vi "HelioScan_3.vi"() -> ()   [LabVIEW 2010]
uses:
  labview_source/controls/update_picture.ctl
  common/xcontrols/XUserDropdown/XUserDropdown/XUserDropdown.xctl
  tools/HelioUpdateMH100803/HelioUpdateMH100803/HelioUpdateMH100803.lvclass
  common/classes/ErrorController/ErrorController/ErrorController.lvclass
  labview_source/type_definitions/clusters/controls_refs.ctl
  components/DAQ/GenericDAQ/GenericDAQ/GenericDAQ.lvclass
  components/ImageAssembler/GenericImageAssembler/GenericImageAssembler/GenericImageAssembler.lvclass
  components/DataCollection/GenericDataCollection/GenericDataCollection/GenericDataCollection.lvclass
  components/Display/GenericDisplay/GenericDisplay/GenericDisplay.lvclass
  components/Analyser/GenericAnalyser/GenericAnalyser/GenericAnalyser.lvclass
  components/ImagingMode/GenericImagingMode/GenericImagingMode/GenericImagingMode.lvclass
  components/Instrument/GenericInstrument/GenericInstrument/GenericInstrument.lvclass
  components/ScanHead/GenericScanHead/GenericScanHead/GenericScanHead.lvclass
  components/Stimulator/GenericStimulator/GenericStimulator/GenericStimulator.lvclass
  components/ExperimentController/GenericExperimentController/GenericExperimentController/GenericExperimentController.lvclass
  components/Stage/GenericStage/GenericStage/GenericStage.lvclass
  <vilib>/Utility/miscctls.llb/LVPointTypeDef.ctl
  components/DataCollection/GenericDataCollection/GenericDataCollection/trigger_enum.ctl
  common/classes/GenericComponent/GenericComponent/GenericComponent.lvclass
  <vilib>/Platform/browser.llb/Open URL in Default Browser (string).vi
  common/classes/ErrorController/ErrorController/class_data.vi
panel:
  in  "button:start_experiment":bool
  in  "button:start_single_sweep":bool
  in  "button:start_focus":bool
  out "saving message":string
  out "progress slider":u8(slide) caption="slider" scale=0.0..11.0
  in  "user":string(xcontrol)
  out "update icon":T1
  in  "file base name":string
  in  "data folder path":path
  in  "notebook":string caption="Notebook"
  in  "exit_button":bool
  in  "objective":string(combo)
  in  "save button":bool
  in  "settings tab":T2(tab)
  in  "imaging mode":string(combo)
  in  "experimental protocol":string(combo)
  in  "stimulator enabled?":bool
  in  "button: task manager":bool
  out "error handler":bool caption="error controller"
  out "experiment controller":bool
  out "imaging mode":bool
  out "scan head":bool
  out "DAQ":bool
  out "image assembler":bool
  out "data collection":bool
  out "display":bool
  out "analyser":bool
  out "stage":bool
  out "stimulator":bool
  out "instrument":bool
  out "Message":string="No Error"
  in  "title":bool caption="HelioScan 3.4.0.23d214112d"
  # "Note: stimulator only works in \"single sweep mode\" and \"experiment mode\"!"
  # "Loaded"
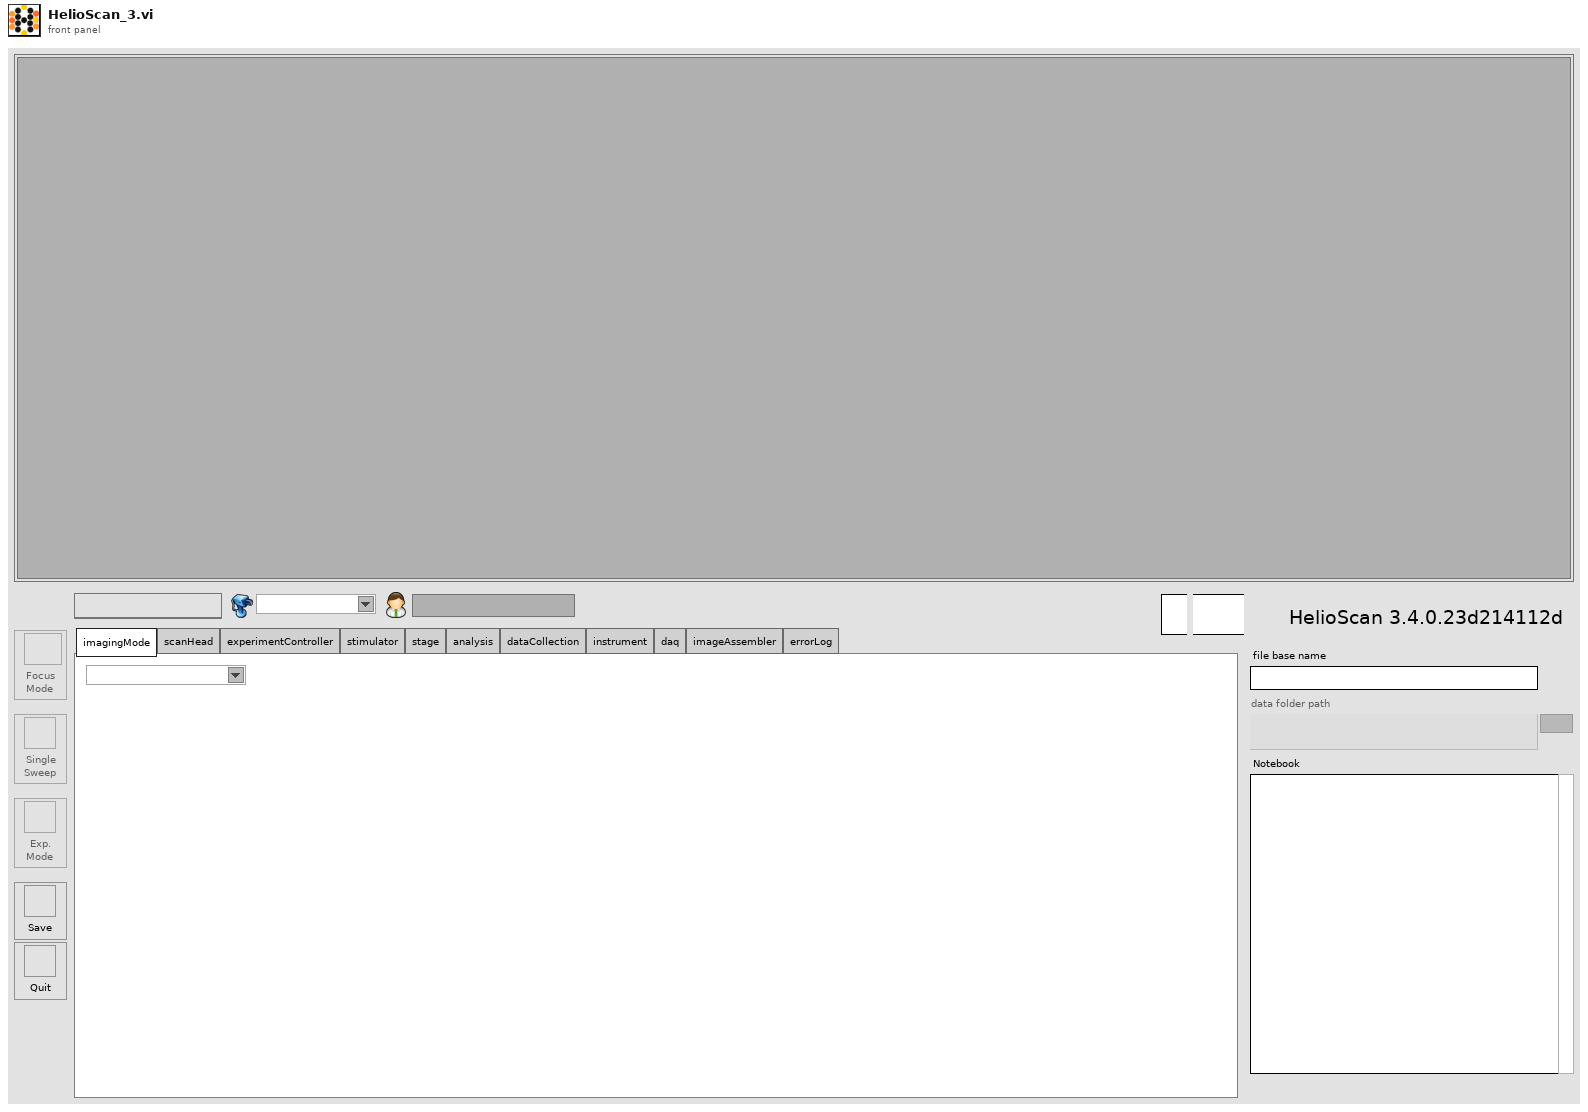
[diagram p1: front panel]
types:
  T1 = typedef "HelioUpdateMH100803.lvclass/update_picture.ctl" = u16
  T2 = enum32{"imagingMode", "scanHead", "experimentController", "stimulator", "stage", "analysis", "dataCollection", "instrument", "daq", "imageAssembler", "errorLog"}
  T3 = typedef "controls_refs.ctl" = cluster{"buttons":cluster{"start_focus":refnum<vi>, "start_single_sweep":refnum<vi>, "start_experiment":refnum<vi>, "save":refnum<vi>, "exit":refnum<vi>}, "tabs":cluster{"main":refnum<vi>, "settings":refnum<vi>}, "subpanels":cluster{"imagingMode":refnum<vi>, "scanHead":refnum<vi>, "display":refnum<vi>, "experimentController":refnum<vi>, "instrument":refnum<vi>, "stage":refnum<vi>, "stimulator":refnum<vi>, "dataCollection":refnum<vi>, "analyser":refnum<vi>, "daq":refnum<vi>, "imageAssembler":refnum<vi>}, "drop-downs":cluster{"imagingMode":refnum<vi>, "experimentalController":refnum<vi>, "objective":refnum<vi>}, "status lights":cluster{"experimentController":refnum<vi>, "imagingMode":refnum<vi>, "scanHead":refnum<vi>, "daq":refnum<vi>, "imageAssembler":refnum<vi>, "dataCollection":refnum<vi>, "display":refnum<vi>, "analyser":refnum<vi>, "stage":refnum<vi>, "stimulator":refnum<vi>, "instrument":refnum<vi>}, "message":refnum<vi>, "stimulator enabled?":refnum<vi>, "saving":cluster{"data folder path":refnum<vi>, "file base name":refnum<vi>, "notebook":refnum<vi>}, "progress bar":refnum<vi>, "update icon":refnum<vi>, "title":refnum<vi>, "main vi":refnum<vi>, "user":refnum<vi>}
  T4 = typedef "LVPointTypeDef.ctl" = cluster{"Horizontal":i16, "Vertical":i16}
  T5 = typedef "GenericDataCollection.lvclass/trigger_enum.ctl" = enum16{"NULL", "save", "reset"}
  T6 = enum8{"Enabled", "Disabled", "Disabled and Grayed Out"}
  T7 = enum32{"Invalid", "Standard", "Closed", "Hidden", "Minimized", "Maximized"}
  T8 = enum16{"focus mode", "single sweep mode", "experiment mode"}
  T9 = typedef "main_trigger_enum.ctl" = enum16{"NULL", "initialise", "terminate", "start", "stop", "change objective", "change experimentController", "change imagingMode", "save notebook", "started saving", "finished saving", "expCtr ready", "expCtr missing", "imgMd ready", "imgMd missing", "scanHd ready", "scanHd missing", "DAQ ready", "DAQ missing", "imgAsm ready", "imgAsm missing", "dataColl ready", "dataColl missing", "display ready", "display missing", "analysr ready", "analysr missing", "instrmnt ready", "instrmnt missing", "stimltr ready", "stimltr missing", "stage ready", "stage missing"}
  T10 = typedef "run_mode_enum.ctl" = enum16{"focus mode", "single sweep mode", "experiment mode"}
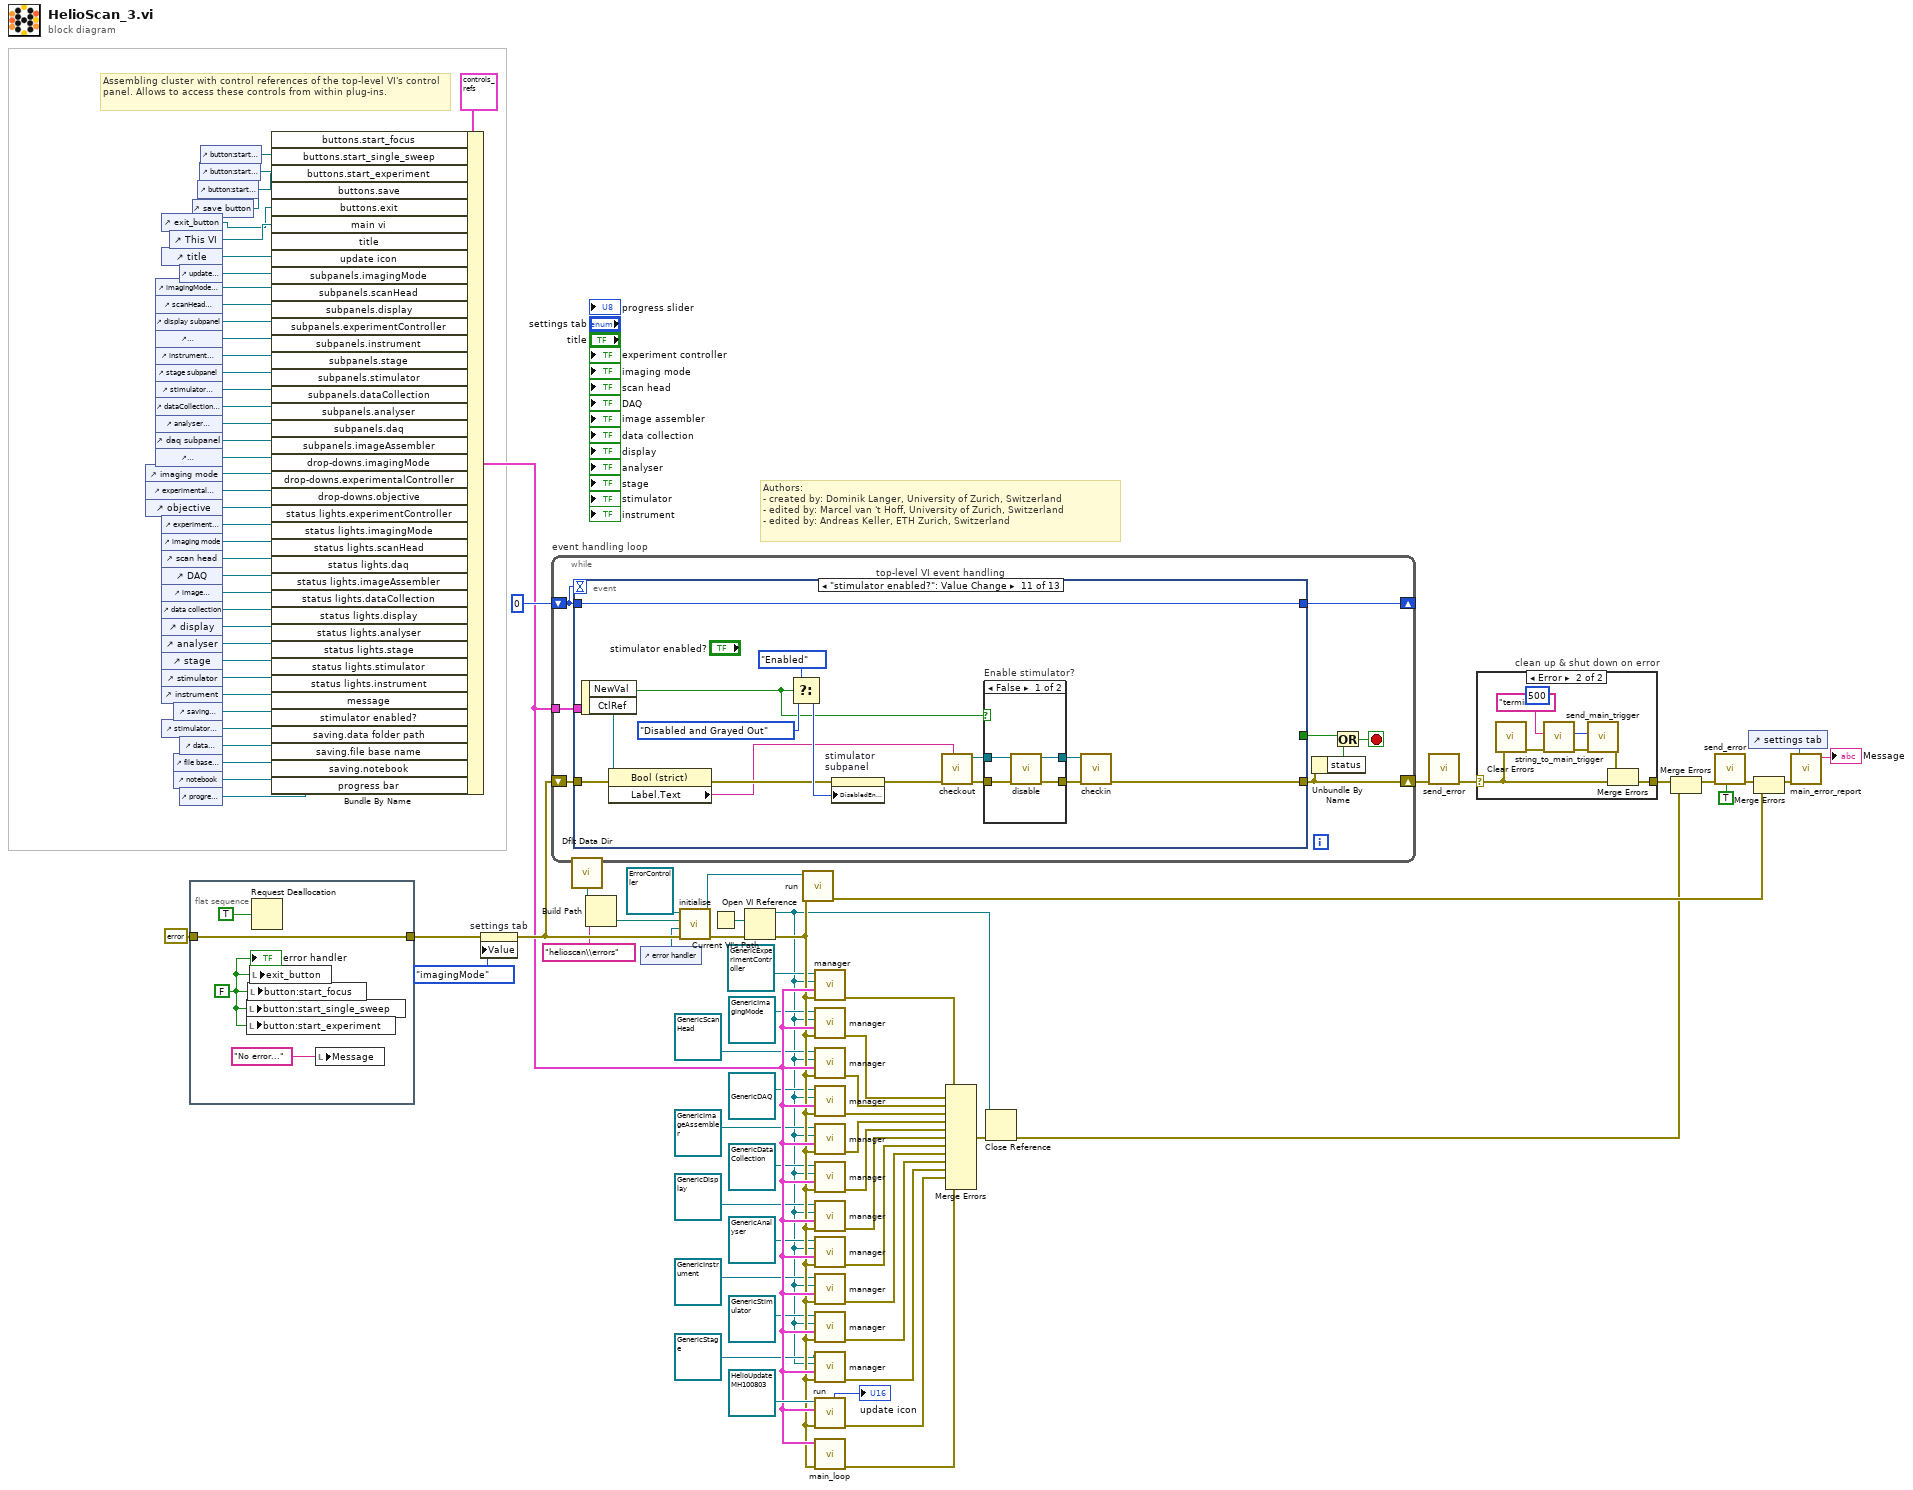
[diagram p0: block diagram]
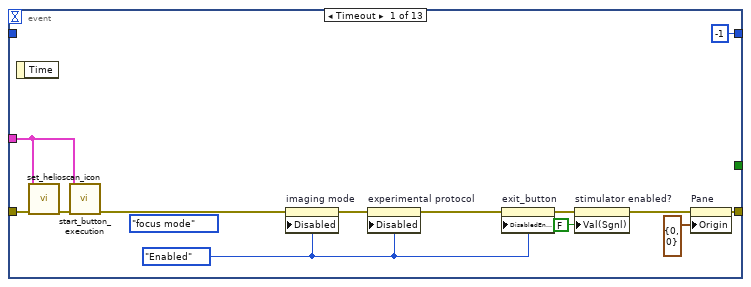
[diagram p3: hidden frame]
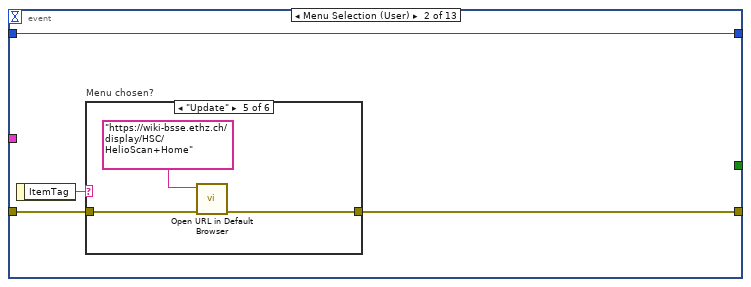
[diagram p4: hidden frame]
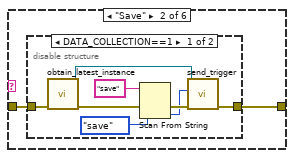
[diagram p6: hidden frame]
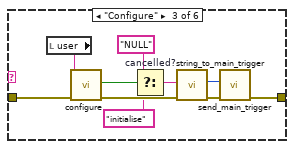
[diagram p8: hidden frame]
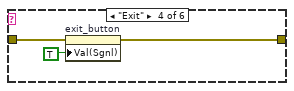
[diagram p9: hidden frame]
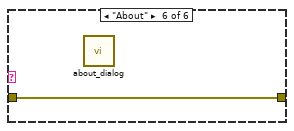
[diagram p10: hidden frame]
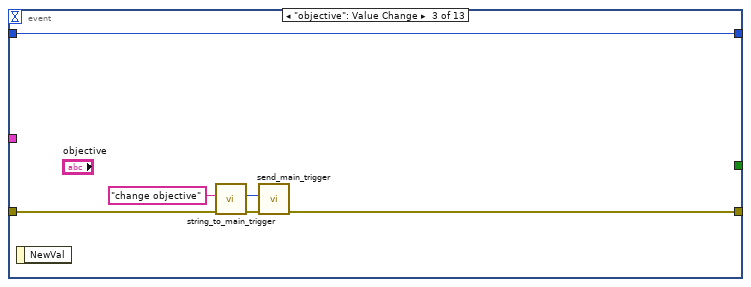
[diagram p11: hidden frame]
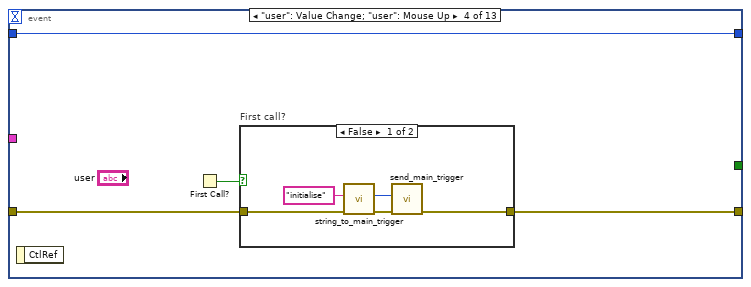
[diagram p12: hidden frame]
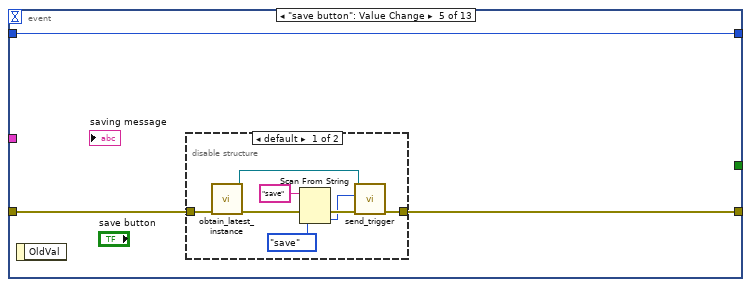
[diagram p14: hidden frame]
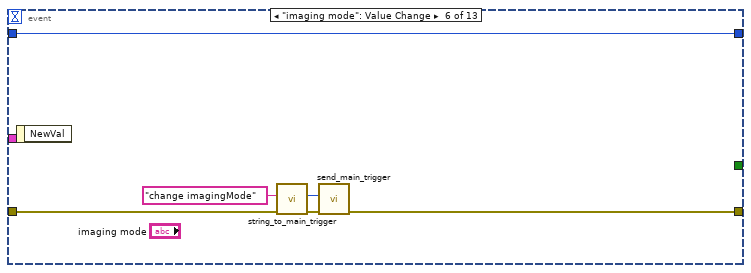
[diagram p16: hidden frame]
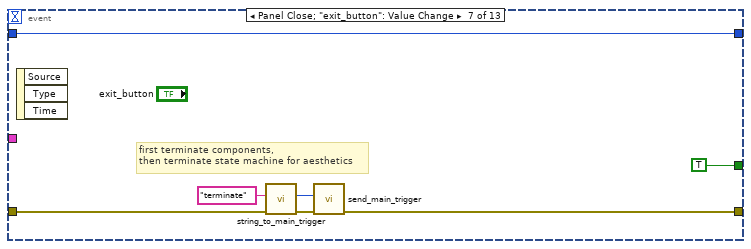
[diagram p17: hidden frame]
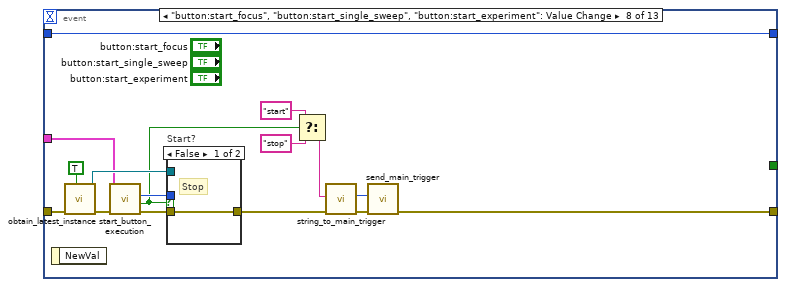
[diagram p18: hidden frame]
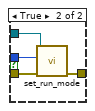
[diagram p19: hidden frame]
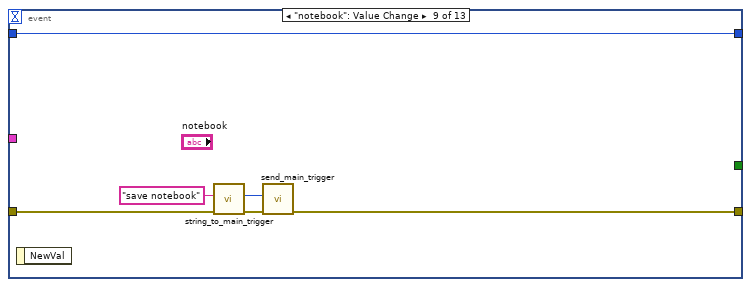
[diagram p20: hidden frame]
diagram:
  # "Authors: \n- created by: Dominik Langer, University of Zurich, Switzerland\n- edited by: Marcel van 't Hoff, University of Zurich, Switzerland\n- edited by: Andreas Keller, ETH Zurich, Switzerland"
  # "Assembling cluster with control references of the top-level VI's control panel. Allows to access these controls from within plug-ins."
  n1 = control-ref of="imaging mode"() -> (w83:refnum<vi>)
  n2 = control-ref of="experimental protocol"() -> (w84:refnum<vi>)
  n3 = control-ref of="objective"() -> (w69:refnum<vi>)
  n4 = control-ref of="imagingMode subpanel"() -> (w63:refnum<vi>)
  n5 = control-ref of="scanHead subpanel"() -> (w94:refnum<vi>)
  n6 = control-ref of="display subpanel"() -> (w90:refnum<vi>)
  n7 = control-ref of="experimentController subpanel"() -> (w91:refnum<vi>)
  n8 = control-ref of="instrument subpanel"() -> (w89:refnum<vi>)
  n9 = control-ref of="stage subpanel"() -> (w87:refnum<vi>)
  n10 = control-ref of="stimulator subpanel"() -> (w86:refnum<vi>)
  n11 = control-ref of="dataCollection subpanel"() -> (w85:refnum<vi>)
  n12 = control-ref of="analyser subpanel"() -> (w82:refnum<vi>)
  n13 = control-ref of="daq subpanel"() -> (w61:refnum<vi>)
  n14 = control-ref of="imageAssembler subpanel"() -> (w62:refnum<vi>)
  n15 = control-ref of="exit_button"() -> (w1:refnum<vi>)
  n16 = control-ref of="title"() -> (w44:refnum<vi>)
  n17 = control-ref of="experiment controller"() -> (w73:refnum<vi>)
  n18 = control-ref of="imaging mode"() -> (w72:refnum<vi>)
  n19 = control-ref of="scan head"() -> (w76:refnum<vi>)
  n20 = control-ref of="DAQ"() -> (w75:refnum<vi>)
  n21 = control-ref of="image assembler"() -> (w74:refnum<vi>)
  n22 = control-ref of="data collection"() -> (w71:refnum<vi>)
  n23 = control-ref of="display"() -> (w77:refnum<vi>)
  n24 = control-ref of="analyser"() -> (w78:refnum<vi>)
  n25 = control-ref of="stage"() -> (w81:refnum<vi>)
  n26 = control-ref of="stimulator"() -> (w80:refnum<vi>)
  n27 = control-ref of="instrument"() -> (w70:refnum<vi>)
  n28 = control-ref of="stimulator enabled?"() -> (w67:refnum<vi>)
  n29 = control-ref of="This VI"() -> (w41:refnum<vi>)
  n30 = control-ref of="saving message"() -> (w45:refnum<vi>)
  n31 = control-ref of="file base name"() -> (w65:refnum<vi>)
  n32 = control-ref of="notebook"() -> (w64:refnum<vi>)
  n33 = control-ref of="update icon"() -> (w43:refnum<vi>)
  n34 = control-ref of="data folder path"() -> (w66:refnum<vi>)
  n35 = control-ref of="progress bar"() -> (w49:refnum<vi>)
  n36 = flat-sequence {
    tunnel: errorcluster {"status"=FALSE, "code"=0, "source"=""} ("error in (no error)") -> [w98]
    tunnel: [w98] -> w7
    frame #0 {
      w95 = FALSE
      n37 = local write "button:start_single_sweep"(w95) -> ()
      n38 = local write "button:start_experiment"(w95) -> ()
      n39 = local write "button:start_focus"(w95) -> ()
      n40 = local write "exit_button"(w95) -> ()
      n41 = Request Deallocation(TRUE ("flag")) -> ()
      n42 = local write "Message"("No error...") -> ()
      "error handler" <- w95
    }
  }
  n43 = control-ref of="save button"() -> (w2:refnum<vi>)
  n44 = control-ref of="button:start_experiment"() -> (w3:refnum<vi>)
  n45 = control-ref of="button:start_single_sweep"() -> (w4:refnum<vi>)
  n46 = control-ref of="button:start_focus"() -> (w5:refnum<vi>)
  n47 = Bundle By Name(cluster=T3 {"buttons"={"start_focus"=refnum, "start_single_sweep"=refnum, "start_experiment"=refnum, "save"=refnum, "exit"=refnum}, "tabs"={"main"=refnum, "settings"=refnum}, "subpanels"={"imagingMode"=refnum, "scanHead"=refnum, "display"=refnum, "experimentController"=refnum, "instrument"=refnum, "stage"=refnum, "stimulator"=refnum, "dataCollection"=refnum, "analyser"=refnum, "daq"=refnum, "imageAssembler"=refnum}, "drop-downs"={"imagingMode"=refnum, "experimentalController"=refnum, "objective"=refnum}, "status lights"={"experimentController"=refnum, "imagingMode"=refnum, "scanHead"=refnum, "daq"=refnum, "imageAssembler"=refnum, "dataCollection"=refnum, "display"=refnum, "analyser"=refnum, "stage"=refnum, "stimulator"=refnum, "instrument"=refnum}, "message"=refnum, "stimulator enabled?"=refnum, "saving"={"data folder path"=refnum, "file base name"=refnum, "notebook"=refnum}, "progress bar"=refnum, "update icon"=refnum, "title"=refnum, "main vi"=refnum, "user"=refnum} ("control references"), "buttons.start_focus"=w5, "buttons.start_single_sweep"=w4, "buttons.start_experiment"=w3, "buttons.save"=w2, "buttons.exit"=w1, "main vi"=w41, "title"=w44, "update icon"=w43, "subpanels.imagingMode"=w63, "subpanels.scanHead"=w94, "subpanels.display"=w90, "subpanels.experimentController"=w91, "subpanels.instrument"=w89, "subpanels.stage"=w87, "subpanels.stimulator"=w86, "subpanels.dataCollection"=w85, "subpanels.analyser"=w82, "subpanels.daq"=w61, "subpanels.imageAssembler"=w62, "drop-downs.imagingMode"=w83, "drop-downs.experimentalController"=w84, "drop-downs.objective"=w69, "status lights.experimentController"=w73, "status lights.imagingMode"=w72, "status lights.scanHead"=w76, "status lights.daq"=w75, "status lights.imageAssembler"=w74, "status lights.dataCollection"=w71, "status lights.display"=w77, "status lights.analyser"=w78, "status lights.stage"=w81, "status lights.stimulator"=w80, "status lights.instrument"=w70, "message"=w45, "stimulator enabled?"=w67, "saving.data folder path"=w66, "saving.file base name"=w65, "saving.notebook"=w64, "progress bar"=w49) -> (w23:T3)
  n48 = property on="settings tab" class="TabCtl (strict)"(error in=w7, "Value"=T2."imagingMode" ("settings tab")) -> (error out=w35:errorcluster)  [unwired: 1 in, 1 out]
  n49 = while "event handling loop" {
    shift-right: [w104] -> _
    shift-left: 0 -> [w105]
    tunnel: w23 -> [w103]
    shift-right: [w102] -> w38
    shift-left: w35 -> [w106]
    stop <- w99 stop-if-true
    n50 = event "top-level VI event handling" shown="[10] \"stimulator enabled?\": Value Change" {
      selector: _ -> [_ _ _ _ _ _ _ _ _ _ _ _ _]
      dyn-events: _ -> [_ _ _ _ _ _ _ _ _ _ _ _ _]
      timeout: w105 -> [_ _ _ _ _ _ _ _ _ _ _ _ _]
      tunnel: [_ _ _ _ _ _ TRUE _ _ _ _ _ _] -> w101
      tunnel: [w117 w120 w157 w161 w170 w185 w191 w195 w219 w225 w234 w256 w262] -> w102
      tunnel: w106 -> [w110 w121 w156 w159 w169 w184 w187 w199 w218 w226 w232 w253 w273]
      tunnel: [-1 w123 w158 w162 w171 w186 w193 w209 w220 w228 w243 w257 w274] -> w104
      tunnel: w105 -> [_ w123 w158 w162 w171 w186 w193 w209 w220 w228 w243 w257 w274]
      tunnel: w103 -> [w108 _ _ _ _ _ _ w196 _ _ _ _ _]
      event Timeout {
        w114 = T6."Enabled" ("Disabled")
        (unwired) T8."focus mode" ("Value (Signaling)")
        n51 = event-data() -> ()  [unwired: 2 out]
        n52 = call "set_helioscan_icon.vi"("error in (no error)"=w110, "reference cluster in"=w108) -> ("error out"=w109:errorcluster)  [unwired: 9 in]
        n53 = call "start_button_execution.vi"("error in (no error)"=w109, "control references"=w108) -> ("error out"=w107:errorcluster)  [unwired: 7 in, 2 out]
        n54 = property on="imaging mode" class="CmbBox"(error in=w107, "Disabled"=w114) -> (error out=w118:errorcluster)  [unwired: 1 in, 1 out]
        n55 = property on="experimental protocol" class="CmbBox"(error in=w118, "Disabled"=w114) -> (error out=w115:errorcluster)  [unwired: 1 in, 1 out]
        n56 = property on="exit_button" class="Bool (strict)"(error in=w115, "DisabledEnum"=w114) -> (error out=w112:errorcluster)  [unwired: 1 in, 1 out]
        n57 = property on="stimulator enabled?" class="Bool (strict)"(error in=w112, "Val(Sgnl)"=FALSE ("stimulator enabled?")) -> (error out=w113:errorcluster)  [unwired: 1 in, 1 out]
        n58 = property on="Pane" class="Pane"(error in=w113, "Origin"=T4 {"Horizontal"=0, "Vertical"=0}) -> (error out=w117:errorcluster)  [unwired: 1 in, 1 out]
      }
      event Menu Selection (User) {
        n59 = event-data() -> ("ItemTag"=w122:string)  [unwired: 1 out]
        n60 = case "Menu chosen?" shown="\"Update\"" w122 {
          tunnel: w121 -> [w124 w126 w145 w148 w151 w152]
          tunnel: [w124 w125 w143 w146 w150 w152] -> w120
          frame Default {
          }
          frame "Save" {
            n61 = disable-structure shown="DATA_COLLECTION==1" {
              disable-tunnel: w126 -> [w133 w135]
              disable-tunnel: [w134 w135] -> w125
              frame condition #0 (active) {
                n62 = call "obtain_latest_instance.vi"("error in (no error)"=w133) -> ("error out"=w130:errorcluster, "GenericDataCollection out"=w132:refnum<class "GenericDataCollection.lvclass">)  [unwired: 1 in, 8 out]
                n63 = Scan From String(input string="save", error in=w130, default 1=trigger_enum."save" ("trigger")) -> (error out=w129:errorcluster, output 1=w128:T5)  [unwired: 2 in, 2 out]
                n64 = call-dynamic "send_trigger.vi"("error in (no error)"=w129, "trigger"=w128, "GenericDataCollection in"=w132) -> ("error out"=w134:errorcluster)  [unwired: 8 out]
              }
              frame condition #1 {
              }
            }
          }
          frame "Configure" {
            n65 = local read "user"() -> (w144:string)
            n66 = call "configure.vi"("error in (no error)"=w145, "user"=w144) -> ("error out"=w141:errorcluster, "cancelled?"=w142:bool)  [unwired: 1 in, 7 out]
            n67 = Select "cancelled?"(t="NULL", s=w142, f="initialise") -> (s? t:f=w137:string)
            n68 = call "string_to_main_trigger.vi"("error in (no error)"=w141, "trigger string"=w137) -> ("error out"=w140:errorcluster, "main trigger"=w136:T9)  [unwired: 8 in]
            n69 = call "send_main_trigger.vi"("error in (no error)"=w140, "trigger"=w136) -> ("error out"=w143:errorcluster)  [unwired: 9 in]
          }
          frame "Exit" {
            n70 = property on="exit_button" class="Bool (strict)"(error in=w148, "Val(Sgnl)"=TRUE) -> (error out=w146:errorcluster)  [unwired: 1 in, 1 out]
          }
          frame "Update" {
            n71 = call-poly <vilib>:"Open URL in Default Browser.vi"("error in (no error)"=w151, "URL"="https://wiki-bsse.ethz.ch/display/HSC/HelioScan+Home") -> ("error out"=w150:errorcluster)  [unwired: 4 in, 1 out]
          }
          frame "About" {
            n72 = call "about_dialog.vi"() -> ()  [unwired: 1 out]
          }
        }
      }
      event "objective": Value Change {
        n73 = event-data() -> ()  [unwired: 2 out]
        n74 = call "string_to_main_trigger.vi"("error in (no error)"=w156, "trigger string"="change objective") -> ("error out"=w155:errorcluster, "main trigger"=w154:T9)  [unwired: 8 in]
        n75 = call "send_main_trigger.vi"("error in (no error)"=w155, "trigger"=w154) -> ("error out"=w157:errorcluster)  [unwired: 9 in]
      }
      event "user": Value Change; "user": Mouse Up {
        n76 = event-data() -> ()  [unwired: 2 out]
        n77 = First Call?() -> (First Call?: T/F=w160:bool)
        n78 = case "First call?" shown="False" w160 {
          tunnel: [w167 w168] -> w161
          tunnel: w159 -> [w166 w168]
          frame False {
            n79 = call "string_to_main_trigger.vi"("error in (no error)"=w166, "trigger string"="initialise") -> ("error out"=w165:errorcluster, "main trigger"=w164:T9)  [unwired: 8 in]
            n80 = call "send_main_trigger.vi"("error in (no error)"=w165, "trigger"=w164) -> ("error out"=w167:errorcluster)  [unwired: 9 in]
          }
          frame True {
          }
        }
      }
      event "save button": Value Change {
        n81 = event-data() -> ()  [unwired: 2 out]
        n82 = disable-structure shown="default" {
          disable-tunnel: [w179 w180] -> w170
          disable-tunnel: w169 -> [w178 w180]
          frame condition #0 (active) {
            n83 = call "obtain_latest_instance.vi"("error in (no error)"=w178) -> ("error out"=w176:errorcluster, "GenericDataCollection out"=w177:refnum<class "GenericDataCollection.lvclass">)  [unwired: 1 in, 8 out]
            n84 = Scan From String(input string="save", error in=w176, default 1=trigger_enum."save" ("trigger")) -> (error out=w175:errorcluster, output 1=w173:T5)  [unwired: 2 in, 2 out]
            n85 = call-dynamic "send_trigger.vi"("error in (no error)"=w175, "trigger"=w173, "GenericDataCollection in"=w177) -> ("error out"=w179:errorcluster)  [unwired: 8 out]
          }
          frame condition #1 {
          }
        }
      }
      event "imaging mode": Value Change {
        n86 = event-data() -> ()  [unwired: 2 out]
        n87 = call "string_to_main_trigger.vi"("error in (no error)"=w184, "trigger string"="change imagingMode") -> ("error out"=w183:errorcluster, "main trigger"=w182:T9)  [unwired: 8 in]
        n88 = call "send_main_trigger.vi"("error in (no error)"=w183, "trigger"=w182) -> ("error out"=w185:errorcluster)  [unwired: 9 in]
      }
      event Panel Close; "exit_button": Value Change {
        # "first terminate components, \nthen terminate state machine for aesthetics"
        n89 = event-data() -> ()  [unwired: 4 out]
        n90 = call "string_to_main_trigger.vi"("error in (no error)"=w187, "trigger string"="terminate") -> ("error out"=w190:errorcluster, "main trigger"=w189:T9)  [unwired: 8 in]
        n91 = call "send_main_trigger.vi"("error in (no error)"=w190, "trigger"=w189) -> ("error out"=w191:errorcluster)  [unwired: 9 in]
      }
      event "button:start_focus", "button:start_single_sweep", "button:start_experiment": Value Change {
        n92 = event-data() -> ()  [unwired: 2 out]
        n93 = call "obtain_latest_instance.vi"("quick, but maybe outdated?"=TRUE, "error in (no error)"=w199) -> ("error out"=w198:errorcluster, "GenericScanMode out"=w208:refnum<class "GenericImagingMode.lvclass">)  [unwired: 8 out]
        n94 = call "start_button_execution.vi"("error in (no error)"=w198, "control references"=w196) -> ("error out"=w197:errorcluster, "start?"=w194:bool, "mode"=w200:T10)  [unwired: 7 in]
        n95 = case "Start?" shown="False" w194 {
          tunnel: w208 -> [_ w214]
          tunnel: [w210 w213] -> w201
          tunnel: w200 -> [_ w212]
          tunnel: w197 -> [w210 w211]
          frame False {
            # "Stop"
          }
          frame True {
            n96 = call-dynamic "set_run_mode.vi"("error in (no error)"=w211, "run mode"=w212, "GenericPlugin in"=w214) -> ("error out"=w213:errorcluster)  [unwired: 8 out]
          }
        }
        n97 = Select(t="start" ("trigger string"), s=w194, f="stop") -> (s? t:f=w203:string)
        n98 = call "string_to_main_trigger.vi"("error in (no error)"=w201, "trigger string"=w203) -> ("error out"=w205:errorcluster, "main trigger"=w206:T9)  [unwired: 8 in]
        n99 = call "send_main_trigger.vi"("error in (no error)"=w205, "trigger"=w206) -> ("error out"=w195:errorcluster)  [unwired: 9 in]
      }
      event "notebook": Value Change {
        n100 = event-data() -> ()  [unwired: 2 out]
        n101 = call "string_to_main_trigger.vi"("error in (no error)"=w218, "trigger string"="save notebook") -> ("error out"=w217:errorcluster, "main trigger"=w216:T9)  [unwired: 8 in]
        n102 = call "send_main_trigger.vi"("error in (no error)"=w217, "trigger"=w216) -> ("error out"=w219:errorcluster)  [unwired: 9 in]
      }
      event "file base name", "data folder path": Value Change {
        n103 = event-data() -> ()  [unwired: 2 out]
        n104 = call-dynamic "set_data_folder_path.vi"("error in (no error)"=w226, "data folder path"="data folder path", "GenericComponent in"=refnum<class "GenericComponent.lvclass"> refnum ("GenericComponent.lvclass")) -> ("error out"=w227:errorcluster, "GenericComponent out"=w222:refnum<class "GenericComponent.lvclass">)  [unwired: 7 out]
        n105 = call-dynamic "set_file_name_base.vi"("error in (no error)"=w227, "file name base"="file base name", "GenericComponent in"=w222) -> ("error out"=w225:errorcluster)  [unwired: 8 out]
      }
      event "stimulator enabled?": Value Change {
        n106 = event-data() -> ("NewVal"=w229:bool, "CtlRef"=w233:refnum<vi>)  [unwired: 1 out]
        n107 = property class="Bool (strict)"(reference=w233, error in=w232) -> (error out=w231:errorcluster, "Label.Text"=w230:string)  [unwired: 1 out]
        n108 = Select(t=T6."Enabled" ("Disabled"), s=w229, f=T6."Disabled and Grayed Out") -> (s? t:f=w241:T6)
        n109 = property on="stimulator\nsubpanel" class="SubPnl"(error in=w231, "DisabledEnum"=w241) -> (error out=w235:errorcluster)  [unwired: 1 in, 1 out]
        n110 = call "checkout.vi"("locked by?"=w230, "error in (no error)"=w235) -> ("error out"=w238:errorcluster, "GenericStimulator out"=w239:refnum<class "GenericStimulator.lvclass">)  [unwired: 8 in]
        n111 = case "Enable stimulator?" shown="False" w229 {
          tunnel: w239 -> [w247 w251]
          tunnel: w238 -> [w246 w250]
          tunnel: [w245 w248] -> w237
          tunnel: [w244 w249] -> w236
          frame False {
            n112 = call-dynamic "disable.vi"("error in (no error)"=w246, "GenericStimulator in"=w247) -> ("error out"=w244:errorcluster, "GenericStimulator out"=w245:refnum<class "GenericStimulator.lvclass">)  [unwired: 8 in]
          }
          frame True {
            n113 = call-dynamic "enable.vi"("error in (no error)"=w250, "GenericStimulator in"=w251) -> ("error out"=w249:errorcluster, "GenericStimulator out"=w248:refnum<class "GenericStimulator.lvclass">)  [unwired: 8 in]
          }
        }
        n114 = call-dynamic "checkin.vi"("error in (no error)"=w236, "GenericStimulator in"=w237) -> ("error out"=w234:errorcluster)  [unwired: 8 in, 1 out]
      }
      event "experimental protocol": Value Change {
        n115 = event-data() -> ()  [unwired: 2 out]
        n116 = call "string_to_main_trigger.vi"("error in (no error)"=w253, "trigger string"="change experimentController") -> ("error out"=w254:errorcluster, "main trigger"=w255:T9)  [unwired: 8 in]
        n117 = call "send_main_trigger.vi"("error in (no error)"=w254, "trigger"=w255) -> ("error out"=w256:errorcluster)  [unwired: 9 in]
      }
      event "button: task manager": Value Change {
        n118 = event-data() -> ()  [unwired: 2 out]
        n119 = Current VI's Path() -> (path=w272:path)
        n120 = call "strip_path_multiple.vi"("error in (no error)"=w273, "number of strips"=2, "path in"=w272) -> ("error out"=w267:errorcluster, "path out"=w270:path)  [unwired: 7 in]
        n121 = Build Path(base path=w270, name or relative path="common\\utilities\\task_manager.vi") -> (appended path=w268:path)
        n122 = Open VI Reference(vi path=w268, error in (no error)=w267) -> (vi reference=w266:refnum<vi>, error out=w265:errorcluster)  [unwired: 4 in]
        n123 = invoke class="VI" method="Run VI"(reference=w266, error in=w265, "Wait until done"=FALSE ("Wait Until Done"), "Auto Dispose Ref"=TRUE ("Auto Dispose Reference")) -> (reference out=w264:refnum<vi>, error out=w263:errorcluster)  [unwired: 1 in, 3 out]
        n124 = invoke class="VI" method="FP.Open"(reference=w264, error in=w263, "Activate"=TRUE ("Activate?"), "State"=T7."Standard") -> (error out=w262:errorcluster)  [unwired: 1 in, 4 out]
      }
    }
    n125 = Unbundle By Name(w102) -> ("status"=w100:bool)
    n126 = Or(x=w101, y=w100) -> (x .or. y?=w99:bool)
  }
  n127 = call <vilib>:"Dflt Data Dir.vi"() -> ("App:Default Data Directory"=w26:path)
  n128 = Build Path(base path=w26, name or relative path="helioscan\\errors") -> (appended path=w24:path)
  n129 = control-ref of="error handler"() -> (w27:refnum<vi>)
  n130 = call-dynamic "initialise.vi"("error in (no error)"=w35, "error boolean"=w27, "error file store path"=w24, "ErrorController in"=refnum<class "ErrorController.lvclass"> refnum) -> ("error out"=w34:errorcluster, "ErrorController out"=w33:refnum<class "ErrorController.lvclass">)  [unwired: 6 in]
  n131 = Current VI's Path() -> (path=w88:path)
  n132 = Open VI Reference(vi path=w88, error in (no error)=w34) -> (vi reference=w10:refnum<vi>, error out=w22:errorcluster)  [unwired: 1 in, 3 out]
  n133 = call "run.vi"("error in (no error)"=w22, "ErrorController in"=w33) -> ("error out"=w32:errorcluster)  [unwired: 8 in, 1 out]
  n134 = call-dynamic "manager.vi"("error in (no error)"=w22, "control references"=w23, "top-level VI ref in"=w10, "GenericToplevelComponent in"=refnum<class "GenericExperimentController.lvclass"> refnum ("GenericExperimentController.lvclass")) -> ("error out"=w50:errorcluster)  [unwired: 5 in, 2 out]
  n135 = call-dynamic "manager.vi"("error in (no error)"=w22, "control references"=w23, "top-level VI ref in"=w10, "GenericToplevelComponent in"=refnum<class "GenericImagingMode.lvclass"> refnum ("GenericImagingMode.lvclass")) -> ("error out"=w53:errorcluster)  [unwired: 5 in, 2 out]
  n136 = call-dynamic "manager.vi"("error in (no error)"=w22, "control references"=w23, "top-level VI ref in"=w10, "GenericToplevelComponent in"=refnum<class "GenericScanHead.lvclass"> refnum ("GenericScanHead.lvclass")) -> ("error out"=w52:errorcluster)  [unwired: 5 in, 2 out]
  n137 = call-dynamic "manager.vi"("error in (no error)"=w22, "control references"=w23, "top-level VI ref in"=w10, "GenericToplevelComponent in"=refnum<class "GenericDAQ.lvclass"> refnum ("GenericDAQ.lvclass")) -> ("error out"=w51:errorcluster)  [unwired: 5 in, 2 out]
  n138 = call-dynamic "manager.vi"("error in (no error)"=w22, "control references"=w23, "top-level VI ref in"=w10, "GenericToplevelComponent in"=refnum<class "GenericImageAssembler.lvclass"> refnum ("GenericImageAssembler.lvclass")) -> ("error out"=w60:errorcluster)  [unwired: 5 in, 2 out]
  n139 = call-dynamic "manager.vi"("error in (no error)"=w22, "control references"=w23, "top-level VI ref in"=w10, "GenericToplevelComponent in"=refnum<class "GenericDataCollection.lvclass"> refnum ("GenericDataCollection.lvclass")) -> ("error out"=w59:errorcluster)  [unwired: 5 in, 2 out]
  n140 = call-dynamic "manager.vi"("error in (no error)"=w22, "control references"=w23, "top-level VI ref in"=w10, "GenericToplevelComponent in"=refnum<class "GenericDisplay.lvclass"> refnum ("GenericDisplay.lvclass")) -> ("error out"=w58:errorcluster)  [unwired: 5 in, 2 out]
  n141 = call-dynamic "manager.vi"("error in (no error)"=w22, "control references"=w23, "top-level VI ref in"=w10, "GenericToplevelComponent in"=refnum<class "GenericAnalyser.lvclass"> refnum ("GenericAnalyser.lvclass")) -> ("error out"=w57:errorcluster)  [unwired: 5 in, 2 out]
  n142 = call-dynamic "manager.vi"("error in (no error)"=w22, "control references"=w23, "top-level VI ref in"=w10, "GenericToplevelComponent in"=refnum<class "GenericInstrument.lvclass"> refnum ("GenericInstrument.lvclass")) -> ("error out"=w56:errorcluster)  [unwired: 5 in, 2 out]
  n143 = call-dynamic "manager.vi"("error in (no error)"=w22, "control references"=w23, "top-level VI ref in"=w10, "GenericToplevelComponent in"=refnum<class "GenericStimulator.lvclass"> refnum ("GenericStimulator.lvclass")) -> ("error out"=w55:errorcluster)  [unwired: 5 in, 2 out]
  n144 = call-dynamic "manager.vi"("error in (no error)"=w22, "control references"=w23, "top-level VI ref in"=w10, "GenericToplevelComponent in"=refnum<class "GenericStage.lvclass"> refnum ("GenericStage.lvclass")) -> ("error out"=w54:errorcluster)  [unwired: 5 in, 2 out]
  n145 = call-dynamic "run.vi"("error in (no error)"=w22, "control references"=w23, "HelioUpdateMH100803 in"=refnum<class "HelioUpdateMH100803.lvclass"> refnum) -> ("error out"=w42:errorcluster, "update out"=→"update icon":T1)  [unwired: 6 in, 1 out]
  n146 = call "main_loop.vi"("error in (no error)"=w22, "control references"=w23) -> ("error out"=w9:errorcluster)  [unwired: 9 in]
  n147 = Merge Errors(w50, w53, w52, w51, w60, w59, w58, w57, w56, w55, w54, w42, w9) -> (w68:errorcluster)
  n148 = Close Reference(reference=w10, error in (no error)=w68) -> (error out=w8:errorcluster)
  n149 = call "send_error.vi"("error in (no error)"=w38) -> ("error out"=w30:errorcluster)  [unwired: 10 in]
  n150 = case "clean up & shut down on error" shown="Error" w30 {
    selector: w30 -> [w275 w281]
    tunnel: [w275 w280] -> w28
    frame No Error {
    }
    frame Error {
      (unwired) u32 500 ("milliseconds to wait")
      n151 = call <vilib>:"Clear Errors.vi"("error in (no error)"=w281) -> ("error out"=w279:errorcluster)  [unwired: 6 in]
      n152 = call "string_to_main_trigger.vi"("error in (no error)"=w279, "trigger string"="terminate") -> ("error out"=w278:errorcluster, "main trigger"=w276:T9)  [unwired: 8 in]
      n153 = call "send_main_trigger.vi"("error in (no error)"=w278, "trigger"=w276) -> ("error out"=w282:errorcluster)  [unwired: 9 in]
      n154 = Merge Errors(w282, w281) -> (w280:errorcluster)
    }
  }
  n155 = Merge Errors(w28, w8) -> (w29:errorcluster)
  n156 = call "send_error.vi"("last error? (F)"=TRUE, "error in (no error)"=w29) -> ("error out"=w37:errorcluster)  [unwired: 9 in]
  n157 = control-ref of="settings tab"() -> (w40:refnum<vi>)
  n158 = Merge Errors(w37, w32) -> (w36:errorcluster)
  n159 = call "main_error_report.vi"("error in"=w36, "TabCtl Refnum"=w40) -> ("message"=→"Message":string)  [unwired: 9 in]
